vi "Tx Inline Wait.vi"(8 "error in (no error)":errorcluster, 11 "Plugin in":refnum<class "Plugin.lvclass">) -> (0 "error out":errorcluster, 3 "Plugin out":refnum<class "Plugin.lvclass">)   [LabVIEW 2017, in "DSF Core.lvlib" / "Plugin.lvclass"]
uses:
  Plugin.lvclass
  Plugin.lvclass/Plugin.ctl
  Transfer Group/Transfer Group.lvclass/Transfer Group.ctl
  Timing/Timing.lvclass/Timing.ctl
  Transfer Group/Read Return FIFO.vi
  Transfer Group/Get Return FIFO.vi
  Transfer Group/Errors.vi
  Transfer Group/Return Timeout Error.vi
  Transfer Group/Transfer Group.lvclass
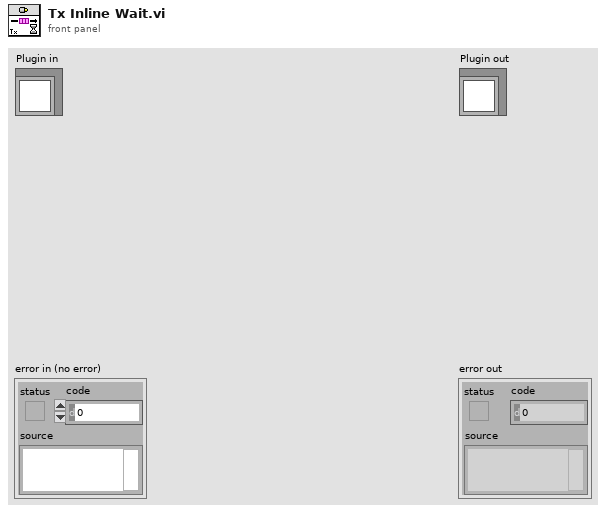
[diagram p1: front panel]
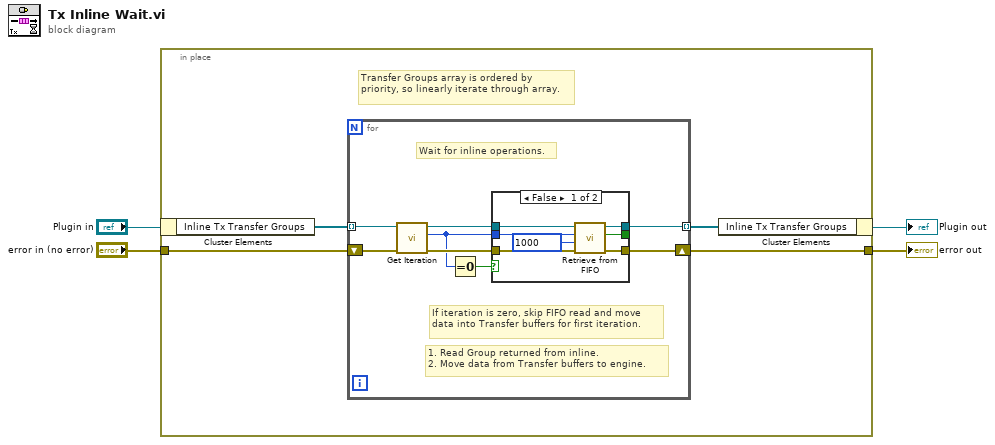
[diagram p0: block diagram]
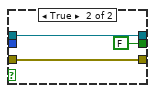
[diagram p2: hidden frame]
diagram:
  n1 = in-place {
    in-place-border: "error in (no error)" -> [w8]
    in-place-border: [w7] -> w3
    # "Transfer Groups array is ordered by priority, so linearly iterate through array."
    n2 = in-place-cluster #1("Plugin in") -> ("Inline Tx Transfer Groups"=w6:refnum<class "Transfer Group.lvclass">[])
    n3 = for {
      tunnel: w6 -> [w13] mode=indexing
      shift-right: [w16] -> w7
      shift-left: w8 -> [w11]
      tunnel: [w15] -> w5 mode=indexing
      # "Wait for inline operations."
      # "If iteration is zero, skip FIFO read and move data into Transfer buffers for first iteration."
      # "1. Read Group returned from inline.\n2. Move data from Transfer buffers to engine."
      n4 = call "Get Iteration.vi"("error in (no error)"=w11, "Transfer Group in"=w13) -> ("error out"=w10:errorcluster, "iteration"=w9:u64, "Transfer Group out"=w12:refnum<class "Transfer Group.lvclass">)  [unwired: 7 in]
      n5 = Equal To 0?(x=w9) -> (x = 0?=w14:bool)
      n6 = case shown="False" w14 {
        tunnel: w10 -> [w23 w25]
        tunnel: [w22 w26] -> w15
        tunnel: [w21 w25] -> w16
        tunnel: w12 -> [w20 w26]
        tunnel: w9 -> [w19 _]
        tunnel: [w18 FALSE ("iteration valid?")] -> _
        frame False {
          n7 = call "Retrieve from FIFO.vi"("error in (no error)"=w23, "timeout in ms (0)"=1000, "expected iteration"=w19, "Transfer Group in"=w20) -> ("error out"=w21:errorcluster, "iteration valid?"=w18:bool, "Transfer Group out"=w22:refnum<class "Transfer Group.lvclass">)  [unwired: 5 in]
        }
        frame True {
        }
      }
    }
    n8 = in-place-cluster #1("Inline Tx Transfer Groups"=w5) -> (→"Plugin out":refnum<class "Plugin.lvclass">)
  }
  "error out" <- w3
